vi "Sine ramps pattern.vi"(8 "Out scale":dbl=1.0, 9 "Out offset":dbl, 10 "Waveform parameters 2":T1={"Start magnitude"=1000.0, "Magnitude increment"=1000.0, "Number of pulses"=8, "Ramp length"=32, "Top  length"=480, "Threshold "=3000, "Processing delay"=240, "Stop after"=1, "Detector window"=480, "Upper limit"=8191, "Lower limit"=-8192} {"Lower limit" format="%d (0x%x)"; "Upper limit" format="%d (0x%x)"; "Detector window" format="%dpts"; "Stop after" format="%d sweep(s)"}) -> (1 "In range?":bool, 2 "Waveform":i16[](array[numeric]) format="%d (0x%x)", 3 "Waveform parameters out":T1={"Start magnitude"=0.0, "Magnitude increment"=0.0, "Number of pulses"=0, "Ramp length"=0, "Top  length"=0, "Threshold "=3000, "Processing delay"=240, "Stop after"=1, "Detector window"=480, "Upper limit"=32767, "Lower limit"=32767} {"Lower limit" format="%d (0x%x)"; "Upper limit" format="%d (0x%x)"; "Detector window" format="%dpts"; "Stop after" format="%d sweep(s)"})   [LabVIEW 2024]
uses:
  Waveform parameters.ctl
panel:
  out "I-V waveform":i16[](graph)
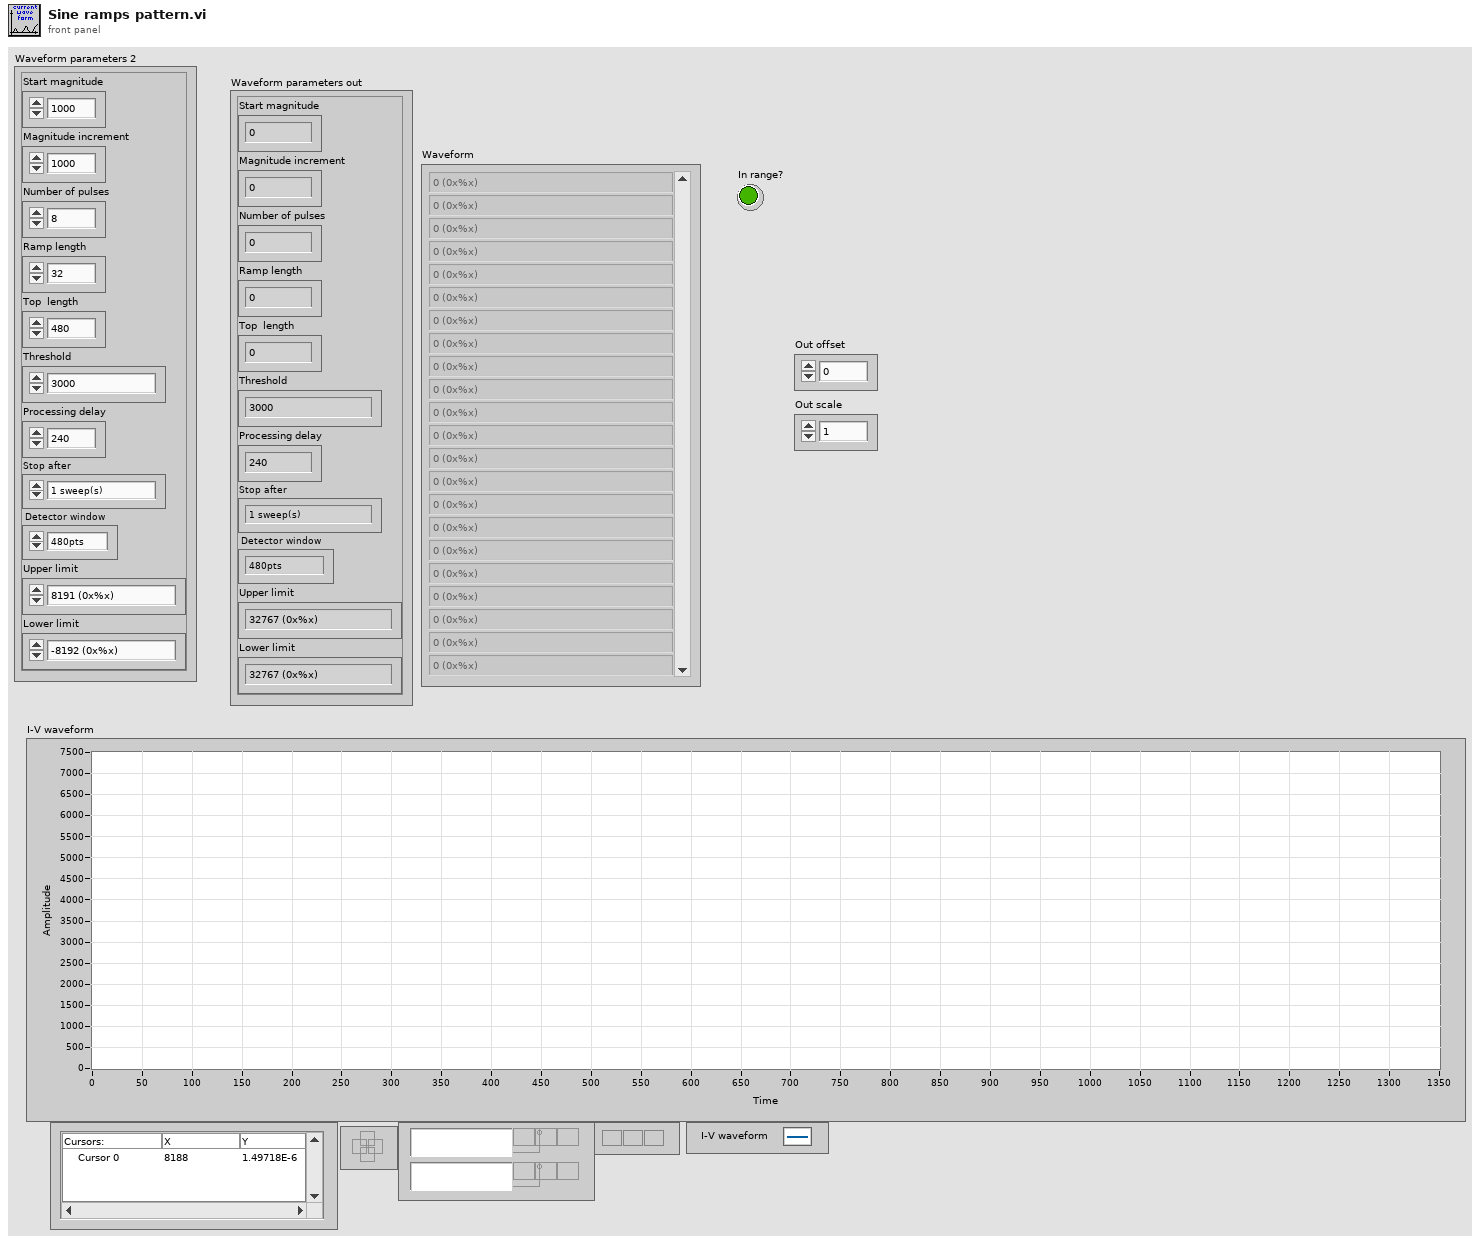
[diagram p1: front panel]
types:
  T1 = typedef "Waveform parameters.ctl" = cluster{"Start magnitude":dbl, "Magnitude increment":dbl, "Number of pulses":i32, "Ramp length":i32, "Top  length":i32, "Threshold ":i32, "Processing delay":u16, "Stop after":u16, "Detector window":i32, "Upper limit":i16, "Lower limit":i16}
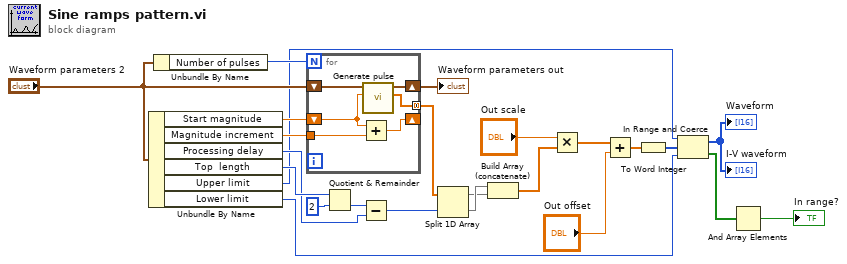
[diagram p0: block diagram]
diagram:
  n1 = Unbundle By Name("Waveform parameters 2") -> ("Start magnitude"=w21:dbl, "Magnitude increment"=w20:dbl, "Processing delay"=w11:u16, "Top  length"=w15:i32, "Upper limit"=w9:i16, "Lower limit"=w8:i16)
  n2 = Unbundle By Name("Waveform parameters 2") -> ("Number of pulses"=w23:i32)
  n3 = for {
    N: w23 -> [_]
    shift-right: [w29] -> w24
    shift-left: "Waveform parameters 2" -> [w30]
    tunnel: [w28] -> w19 mode=concatenating
    shift-right: [w25] -> _
    shift-left: w21 -> [w27]
    tunnel: w20 -> [w26]
    n4 = Add(x=w27, y=w26) -> (x+y=w25:dbl)
    n5 = call "Generate pulse.vi"("Pulse magnitude"=w27, "Waveform parameters"=w30) -> ("Data out"=w28:dbl[], "Waveform parameters out"=w29:T1)  [unwired: 8 in]
  }
  "Waveform parameters out" <- w24
  n6 = Quotient & Remainder(x=w15, y=2) -> (floor(x/y)=w12:i32)  [unwired: 1 out]
  n7 = Subtract(x=w12, y=w11) -> (x-y=w13:i32)
  n8 = Split 1D Array(array=w19, index=w13) -> (first subarray=w16:dbl[], second subarray=w17:dbl[])
  n9 = Build Array (concatenate)(w17, w16) -> (w18:dbl[])
  n10 = Multiply(x="Out scale", y=w18) -> (x*y=w4:dbl[])
  n11 = Add(x=w4, y="Out offset") -> (x+y=w2:dbl[])
  n12 = To Word Integer(number=w2) -> (16bit integer=w10:i16[])
  n13 = In Range and Coerce(upper limit=w9, x=w10, lower limit=w8) -> (coerced(x)=→"I-V waveform" →"Waveform":i16[], In Range?=w6:bool[])
  n14 = And Array Elements(Boolean array=w6) -> (logical AND=→"In range?":bool)
